vi "path_visa_write.vi"(8 "y":i32[](array[numeric]), 11 "x":i32[](array[numeric])) -> (2 "写入缓冲区":string)   [LabVIEW 2016]
uses:
  <vilib>/Instr/_visa.llb/VISA Configure Serial Port (Instr).vi
panel:
  in  "串口配置":T1={"波特率"=115200, "奇偶校验位"=0, "停止位"=10, "流控制"=0, "数据位"=8} {"数据位" items=["8"=8]; "流控制" items=["无"=0, "XON/XOFF"=1, "RTS/CTS"=2, "DTR/DSR"=4]; "停止位" items=["1.0"=10, "2.0"=15, "3.0"=20]; "奇偶校验位" items=["None"]; "波特率" items=["115200"=115200]}
  in  "VISA资源名称":refnum<visa-resource-name>
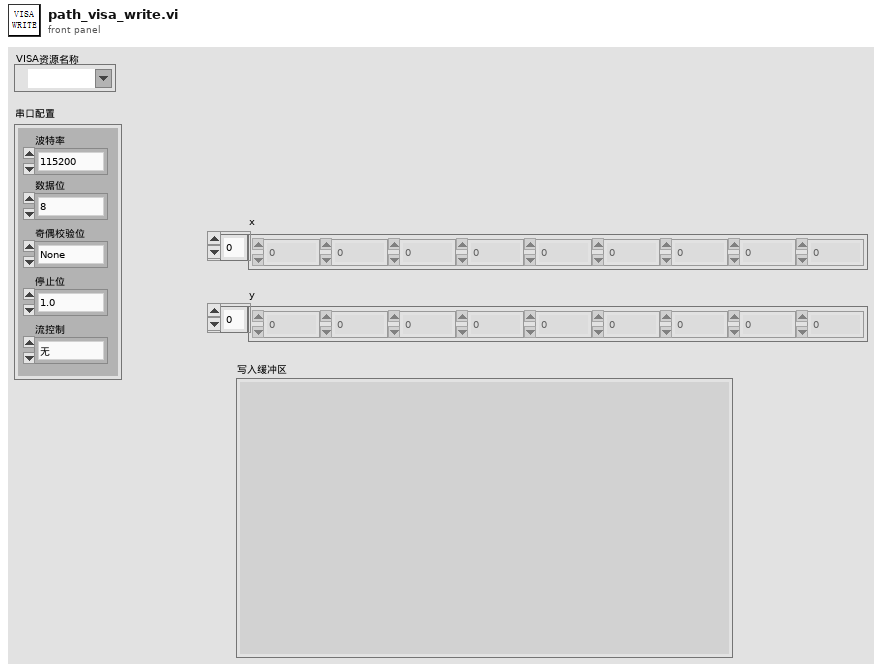
[diagram p1: front panel]
types:
  T1 = cluster{"波特率":u32, "奇偶校验位":u16, "停止位":u16, "流控制":u16, "数据位":u32}
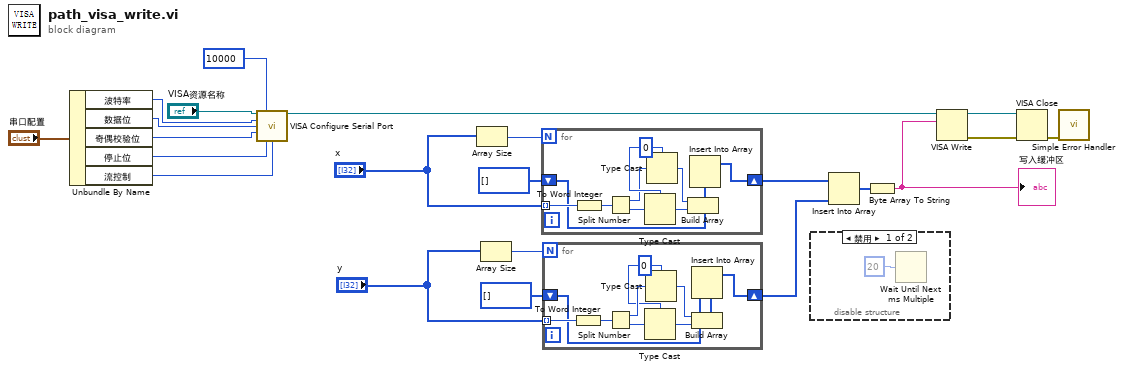
[diagram p0: block diagram]
diagram:
  n1 = Unbundle By Name("串口配置") -> ("波特率"=w20:u32, "数据位"=w19:u32, "奇偶校验位"=w18:u16, "停止位"=w17:u16, "流控制"=w16:u16)
  n2 = call-poly "VISA Configure Serial Port"("VISA resource name"="VISA资源名称", "timeout (10sec)"=u32 10000, "baud rate (9600)"=w20, "data bits (8)"=w19, "parity (0:none)"=w18, "stop bits (10: 1 bit)"=w17, "flow control (0:none)"=w16) -> ("VISA resource name out"=w15:refnum<visa-resource-name>)  [unwired: 7 in, 1 out]
  n3 = Array Size(array="x") -> (size(s)=w8:i32)
  n4 = Array Size(array="y") -> (size(s)=w5:i32)
  n5 = for {
    N: w8 -> [_]
    tunnel: "x" -> [w26] mode=indexing
    shift-right: [w25] -> w1
    shift-left: i32[] [] -> [w24]
    w29 = u8 0
    n6 = To Word Integer(number=w26) -> (16bit integer=w27:i16)
    n7 = Split Number(x=w27) -> (hi(x)=w28:u8, lo(x)=w30:u8)
    n8 = Type Cast(type=w29, x=w30) -> (*(type *) &x=w32:u8)
    n9 = Type Cast(type=w29, x=w28) -> (*(type *) &x=w31:u8)
    n10 = Build Array(w31, w32) -> (w23:u8[])
    n11 = Insert Into Array(array=w24, new element=w23) -> (w25:i32[])  [unwired: 1 in]
  }
  n12 = for {
    N: w5 -> [_]
    tunnel: "y" -> [w37] mode=indexing
    shift-right: [w36] -> w3
    shift-left: i32[] [] -> [w35]
    w33 = u8 0
    n13 = To Word Integer(number=w37) -> (16bit integer=w38:i16)
    n14 = Split Number(x=w38) -> (hi(x)=w39:u8, lo(x)=w40:u8)
    n15 = Type Cast(type=w33, x=w40) -> (*(type *) &x=w42:u8)
    n16 = Type Cast(type=w33, x=w39) -> (*(type *) &x=w41:u8)
    n17 = Build Array(w41, w42) -> (w34:u8[])
    n18 = Insert Into Array(array=w35, new element=w34) -> (w36:i32[])  [unwired: 1 in]
  }
  n19 = disable-structure shown="禁用" {
    frame Disabled {
      n20 = Wait Until Next ms Multiple(millisecond multiple=u32 20 ("毫秒倍数")) -> ()  [unwired: 1 out]
    }
    frame Enabled {
    }
  }
  n21 = Insert Into Array(array=w1, new element=w3) -> (w2:i32[])  [unwired: 1 in]
  n22 = Byte Array To String(unsigned byte array=w2) -> (string=w10:string)
  "写入缓冲区" <- w10
  n23 = VISA Write(VISA resource name=w15, write buffer=w10) -> (VISA resource name out=w12:refnum<visa-resource-name>, error out=w11:errorcluster)  [unwired: 1 in, 1 out]
  n24 = VISA Close(VISA resource name=w12, error in (no error)=w11) -> (error out=w13:errorcluster)
  n25 = call <vilib>:"Simple Error Handler.vi"("error in (no error)"=w13) -> ()  [unwired: 4 in, 5 out]
